vi "ni579x Read EEPROM Header.vi"(0 "Register Bus":refnum<class "ni579x Register Bus v1 Host.lvclass">=refnum, 1 "scope":string(combo)="characterization data eeprom", 5 "start address":u32 format="%x", 11 "Error In":errorcluster) -> (4 "Register Bus (out)":refnum<class "ni579x Register Bus v1 Host.lvclass">, 6 "EEPROM Header":T1 {"Product Code" format="%x"; "Checksum" format="%x"}, 15 "Error Out":errorcluster)   [LabVIEW 2013]
uses:
  <instrlib>/ni579x/Register Bus/v1/Host/ni579x Register Bus v1 Host.lvclass
  <instrlib>/ni579x/Config/v1/Shared/Types/EEPROM/ni579x EEPROM Header.ctl
  <instrlib>/ni579x/Config/v1/Shared/Conversions/From Byte Array (U16).vi
  <instrlib>/ni579x/Config/v1/Shared/Conversions/From Byte Array (U32).vi
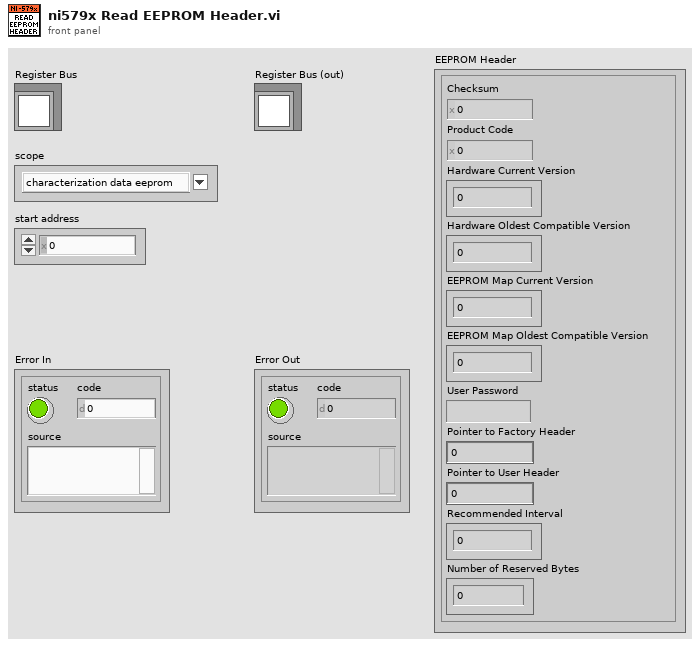
[diagram p1: front panel]
types:
  T1 = typedef "ni579x EEPROM Header.ctl" = cluster{"Checksum":u32, "Product Code":u16, "Hardware Current Version":u16, "Hardware Oldest Compatible Version":u16, "EEPROM Map Current Version":u16, "EEPROM Map Oldest Compatible Version":u16, "User Password":string, "Pointer to Factory Header":u32, "Pointer to User Header":u32, "Recommended Interval":u16, "Number of Reserved Bytes":i32}
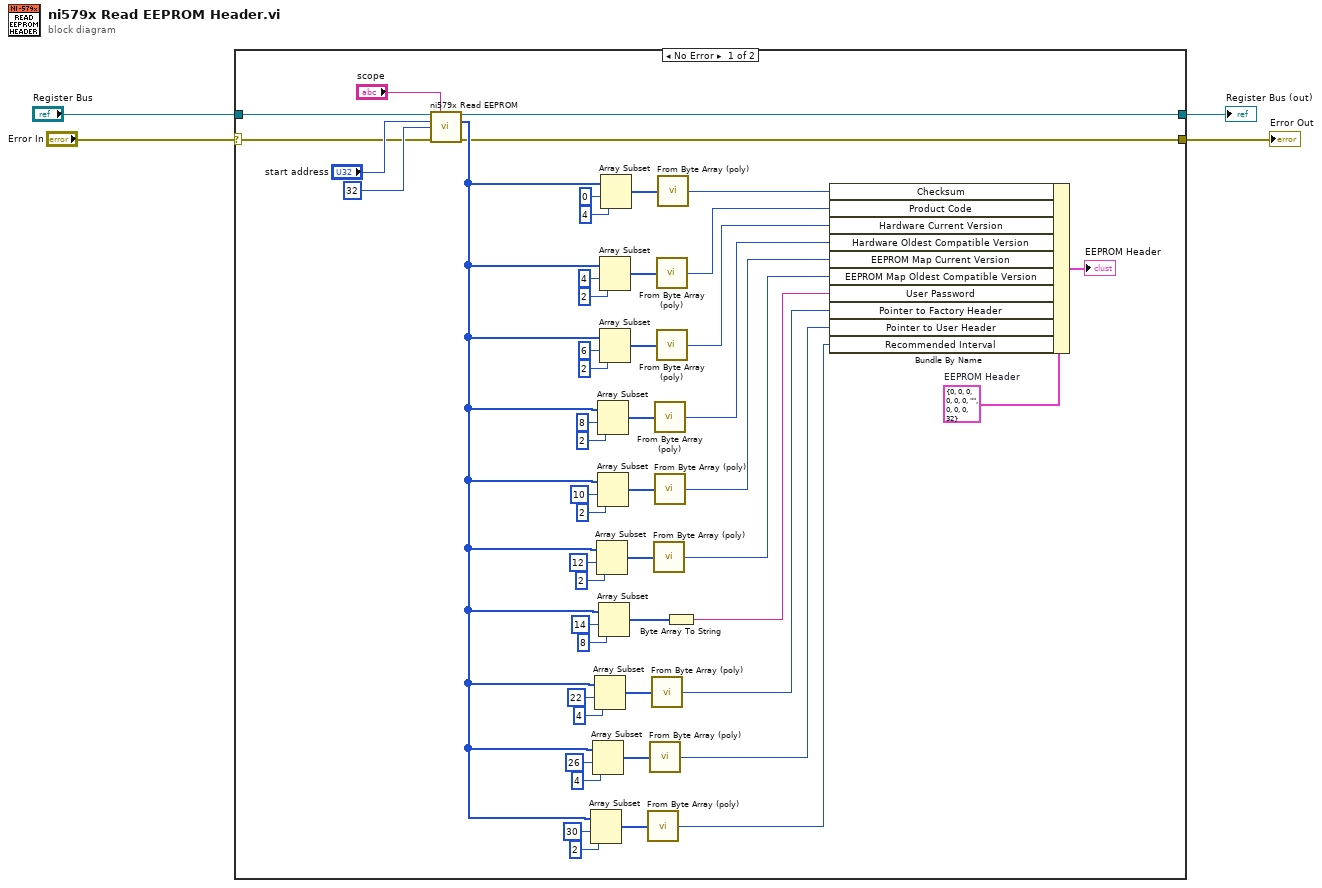
[diagram p0: block diagram]
diagram:
  n1 = case shown="No Error" "Error In" {
    selector: "Error In" -> [w51 w56]
    tunnel: [w8 w56] -> w3
    tunnel: "Register Bus" -> [w52 w55]
    tunnel: [w9 w55] -> w1
    frame No Error {
      w6 = T1 {"Checksum"=0, "Product Code"=0, "Hardware Current Version"=0, "Hardware Oldest Compatible Version"=0, "EEPROM Map Current Version"=0, "EEPROM Map Oldest Compatible Version"=0, "User Password"="", "Pointer to Factory Header"=0, "Pointer to User Header"=0, "Recommended Interval"=0, "Number of Reserved Bytes"=32}  # EEPROM Header
      n2 = call <instrlib>:"ni579x Read EEPROM.vi"("Register Bus"=w52, "scope"="scope", "start address"="start address", "size"=u32 32, "Error In"=w51) -> ("Register Bus (out)"=w9:refnum<class "ni579x Register Bus v1 Host.lvclass">, "data"=w13:u8[], "Error Out"=w8:errorcluster)  [unwired: 8 in]
      n3 = Array Subset(array=w13, index=30, length=2) -> (w14:u8[])
      n4 = Array Subset(array=w13, index=26, length=4) -> (w19:u8[])
      n5 = Array Subset(array=w13, index=22, length=4) -> (w20:u8[])
      n6 = Array Subset(array=w13, index=12, length=2) -> (w28:u8[])
      n7 = Array Subset(array=w13, index=8, length=2) -> (w33:u8[])
      n8 = Array Subset(array=w13, index=10, length=2) -> (w38:u8[])
      n9 = Array Subset(array=w13, index=14, length=8) -> (w24:u8[])
      n10 = Array Subset(array=w13, index=4, length=2) -> (w46:u8[])
      n11 = Array Subset(array=w13, index=6, length=2) -> (w41:u8[])
      n12 = Array Subset(array=w13, index=0, length=4) -> (w48:u8[])
      n13 = call-poly <instrlib>:"From Byte Array (poly).vi"("byte array in"=w14) -> ("element out"=w10:u16)
      n14 = call-poly <instrlib>:"From Byte Array (poly).vi"("byte array in"=w19) -> ("element out"=w11:u32)
      n15 = call-poly <instrlib>:"From Byte Array (poly).vi"("byte array in"=w20) -> ("element out"=w12:u32)
      n16 = call-poly <instrlib>:"From Byte Array (poly).vi"("byte array in"=w28) -> ("element out"=w27:u16)
      n17 = call-poly <instrlib>:"From Byte Array (poly).vi"("byte array in"=w33) -> ("element out"=w32:u16)
      n18 = call-poly <instrlib>:"From Byte Array (poly).vi"("byte array in"=w38) -> ("element out"=w31:u16)
      n19 = call-poly <instrlib>:"From Byte Array (poly).vi"("byte array in"=w46) -> ("element out"=w40:u16)
      n20 = call-poly <instrlib>:"From Byte Array (poly).vi"("byte array in"=w41) -> ("element out"=w39:u16)
      n21 = call-poly <instrlib>:"From Byte Array (poly).vi"("byte array in"=w48) -> ("element out"=w47:u32)
      n22 = Byte Array To String(unsigned byte array=w24) -> (string=w23:string)
      n23 = Bundle By Name(cluster=w6, "Checksum"=w47, "Product Code"=w40, "Hardware Current Version"=w39, "Hardware Oldest Compatible Version"=w32, "EEPROM Map Current Version"=w31, "EEPROM Map Oldest Compatible Version"=w27, "User Password"=w23, "Pointer to Factory Header"=w12, "Pointer to User Header"=w11, "Recommended Interval"=w10) -> (→"EEPROM Header":T1)
    }
    frame Error {
    }
  }
  "Register Bus (out)" <- w1
  "Error Out" <- w3
